vi "Variant to DTItem.vi"(8 "error in (no error)":errorcluster, 10 "datatype":T1, 11 "element":variant) -> (0 "error out":errorcluster, 3 "DTItem .NET Refnum out":refnum<k24>)   [LabVIEW 2016, in "DataGrid.lvlib" / "DataTable.lvclass"]
uses:
  <userlib>/LabVIEWdotNetDataGrid/source/DataTable/DataTable.lvclass
  <userlib>/LabVIEWdotNetDataGrid/source/GridColumn/ColumnType.ctl
  <userlib>/LabVIEWdotNetDataGrid/source/GridColumn/GridColumn.lvclass
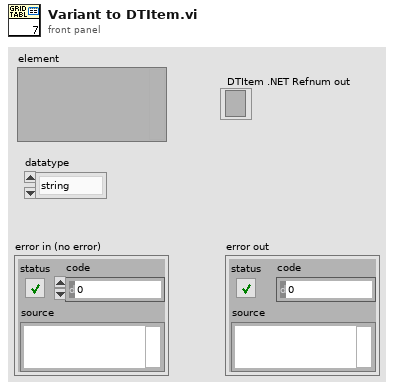
[diagram p1: front panel]
types:
  T1 = typedef "DataGrid.lvlib/GridColumn.lvclass/ColumnType.ctl" = enum16{"string", "image", "check", "numeric", "timestamp", "button", "combo", "link"}
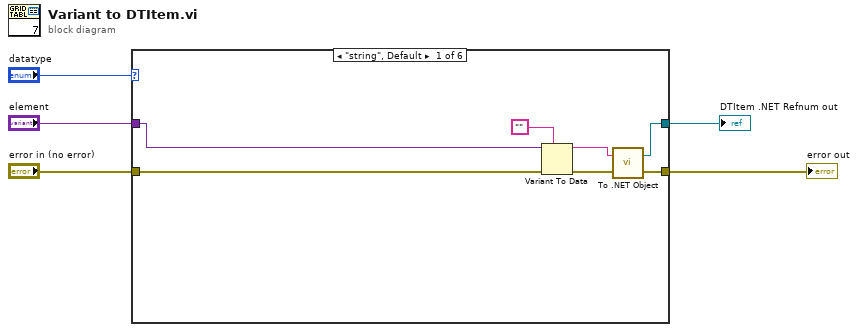
[diagram p0: block diagram]
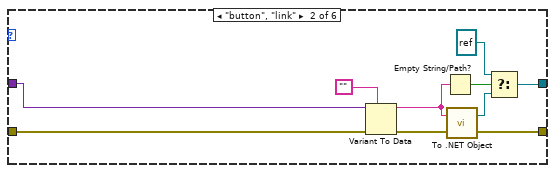
[diagram p2: hidden frame]
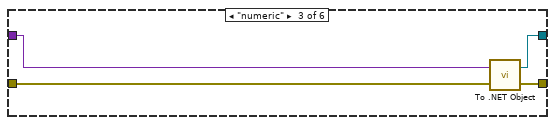
[diagram p3: hidden frame]
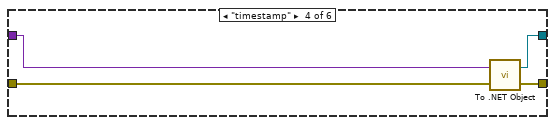
[diagram p4: hidden frame]
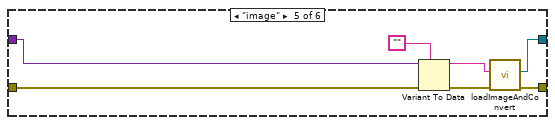
[diagram p5: hidden frame]
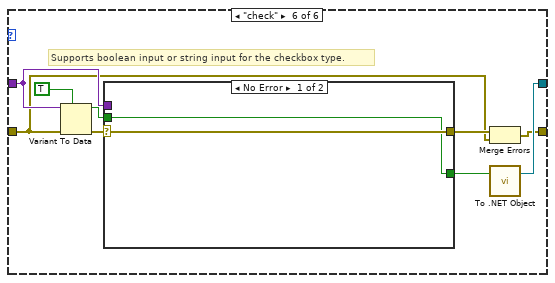
[diagram p6: hidden frame]
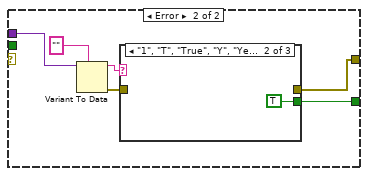
[diagram p7: hidden frame]
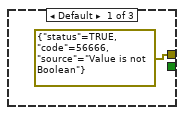
[diagram p8: hidden frame]
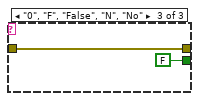
[diagram p9: hidden frame]
diagram:
  n1 = case shown="\"string\", Default" "datatype" {
    tunnel: "element" -> [w9 w19 w24 w28 w33 w41]
    tunnel: [w8 w16 w25 w29 w37 w46] -> w2
    tunnel: "error in (no error)" -> [w12 w22 w23 w27 w35 w39]
    tunnel: [w10 w20 w26 w30 w36 w38] -> w4
    frame "string", Default {
      n2 = Variant To Data(error in=w12, type="", Variant=w9) -> (data=w7:string, error out=w11:errorcluster)
      n3 = call <vilib>:"To .NET Object.vi"("error in (no error)"=w11, "anything"=w7) -> ("error out"=w10:errorcluster, ".NET object"=w8:refnum<k24>)
    }
    frame "button", "link" {
      n4 = Variant To Data(error in=w22, type="", Variant=w19) -> (data=w13:string, error out=w21:errorcluster)
      n5 = Empty String/Path?(string/path=w13) -> (empty?=w18:bool)
      n6 = call <vilib>:"To .NET Object.vi"("error in (no error)"=w21, "anything"=w13) -> ("error out"=w20:errorcluster, ".NET object"=w17:refnum<k24>)
      n7 = Select(t=refnum<k24> refnum, s=w18, f=w17) -> (s? t:f=w16:refnum<k24>)
    }
    frame "numeric" {
      n8 = call <vilib>:"To .NET Object.vi"("error in (no error)"=w23, "anything"=w24) -> ("error out"=w26:errorcluster, ".NET object"=w25:refnum<k24>)
    }
    frame "timestamp" {
      n9 = call <vilib>:"To .NET Object.vi"("error in (no error)"=w27, "anything"=w28) -> ("error out"=w30:errorcluster, ".NET object"=w29:refnum<k24>)
    }
    frame "image" {
      n10 = Variant To Data(error in=w35, type="", Variant=w33) -> (data=w31:string, error out=w34:errorcluster)
      n11 = call <userlib>:"loadImageAndConvert.vi"("error in (no error)"=w34, "name or relative path"=w31) -> ("error out"=w36:errorcluster, ".NET object"=w37:refnum<k24>)  [unwired: 8 in]
    }
    frame "check" {
      # "Supports boolean input or string input for the checkbox type."
      n12 = Variant To Data(error in=w39, type=TRUE, Variant=w41) -> (data=w42:bool, error out=w43:errorcluster)
      n13 = case shown="No Error" w43 {
        selector: w43 -> [w48 _]
        tunnel: [w47 w54] -> w45
        tunnel: [w48 w49] -> w40
        tunnel: w42 -> [w47 _]
        tunnel: w41 -> [_ w52]
        frame No Error {
        }
        frame Error {
          n14 = Variant To Data(type="", Variant=w52) -> (data=w53:string, error out=w50:errorcluster)  [unwired: 1 in]
          n15 = case shown="\"1\", \"T\", \"True\", \"Y\", \"Yes\"" w53 {
            tunnel: [_ TRUE FALSE] -> w54
            tunnel: w50 -> [_ _ w57]
            tunnel: [errorcluster {"status"=TRUE, "code"=56666, "source"="Value is not Boolean"} ("error out") _ w57] -> w49
            frame Default {
            }
            frame "1", "T", "True", "Y", "Yes" {
            }
            frame "0", "F", "False", "N", "No" {
            }
          }
        }
      }
      n16 = Merge Errors(w40, w39) -> (w38:errorcluster)
      n17 = call <vilib>:"To .NET Object.vi"("anything"=w45) -> (".NET object"=w46:refnum<k24>)  [unwired: 1 in, 1 out]
    }
  }
  "error out" <- w4
  "DTItem .NET Refnum out" <- w2
